vi "ConnectedStatusToSLServer.vi"() -> ()   [LabVIEW 2020]
doc: "This VI connects to the SystemLink server and writes two tag values: \nTrue to \"SERVER_NAME.System.Connected\"\nTimestamp of Start Time to \"SERVER_NAME.System.StartTime\""
uses:
  <vilib>/Skyline/Tag/Shared/typedefs/DataType.ctl
  StateStartTimeUpdate.ctl
  <vilib>/Skyline/Configuration/Configuration HTTP_class/NI Skyline Configuration HTTP.lvclass/NI Skyline Configuration HTTP.ctl
  <vilib>/Skyline/Configuration/Configuration HTTP_class/Open Configuration HTTP.vi
  <vilib>/Skyline/Configuration/HTTP/Open Configuration (Desktop).vi
  <vilib>/Skyline/Tag/Wrapper/Wrapper HTTP_class/Open Tag HTTP.vi
  <vilib>/Skyline/Tag/Wrapper/Wrapper_class/Write Tag (Boolean).vi
  <vilib>/Skyline/Tag/Wrapper/Wrapper_class/Delete Tag (Single).vi
  <vilib>/Skyline/Tag/Wrapper/Wrapper_class/Write Tag (Timestamp).vi
  <vilib>/nisyscfg/Close (System).vi
  <vilib>/Skyline/Configuration/Configuration HTTP_class/NI Skyline Configuration HTTP.lvclass
  <vilib>/Skyline/Configuration/Configuration_class/NI Skyline Configuration.lvclass
  <vilib>/Skyline/Tag/Wrapper/Wrapper_class/NI Skyline Tag.lvclass
  <vilib>/Skyline/Tag/Wrapper/Wrapper HTTP_class/NI Skyline Tag HTTP.lvclass
  <vilib>/Skyline/Tag/Shared/NI Skyline Tag.lvlib
  <vilib>/Skyline/Utilities/NI Skyline Utilities.lvlib
  <vilib>/nisyscfg/nisyscfg.lvlib
  <resource>/objmgr/nisysapi.rc
panel:
  in  "stop":bool
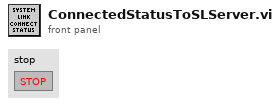
[diagram p1: front panel]
types:
  T1 = typedef "StateStartTimeUpdate.ctl" = enum16{"Init", "UpdateStartTime", "CleanUp"}
  T2 = typedef "NI Skyline Tag.lvlib/DataType.ctl" = enum32{"Double", "I32", "String", "Boolean", "U64", "Timestamp"}
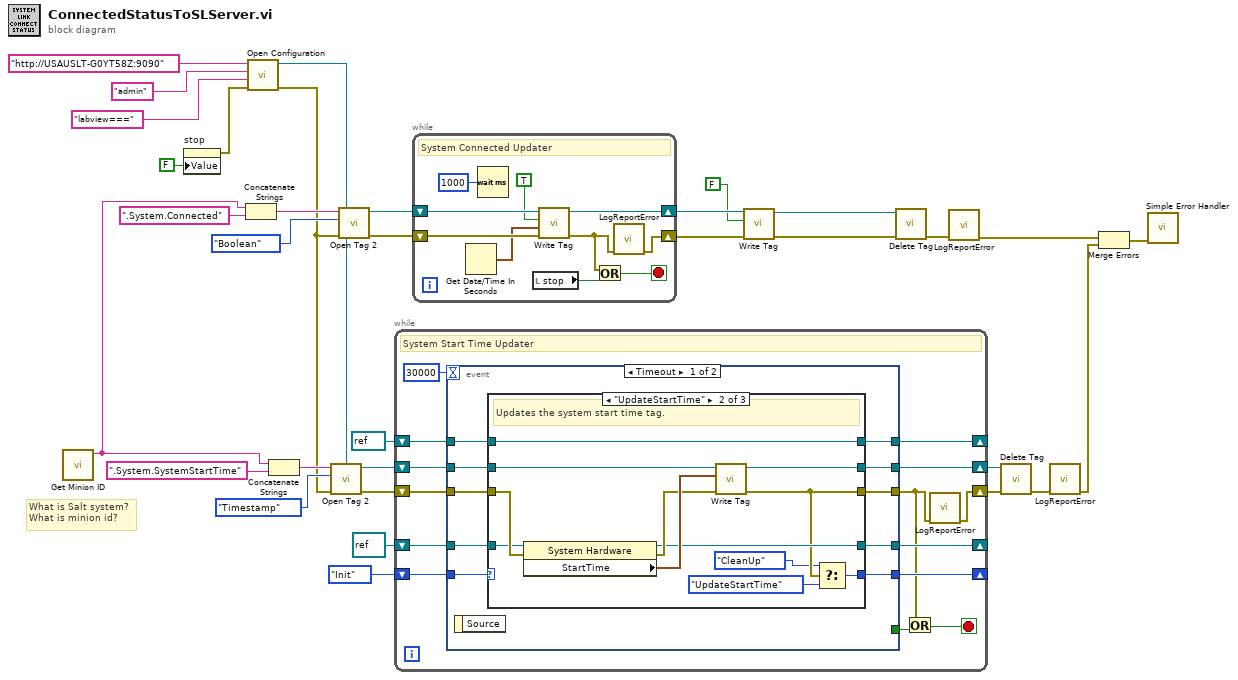
[diagram p0: block diagram]
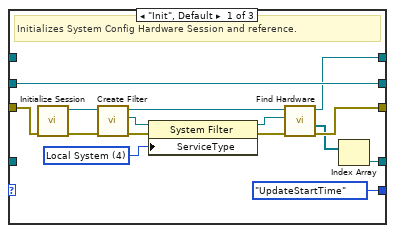
[diagram p2: hidden frame]
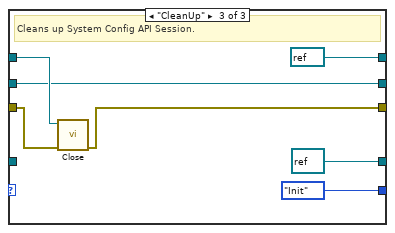
[diagram p3: hidden frame]
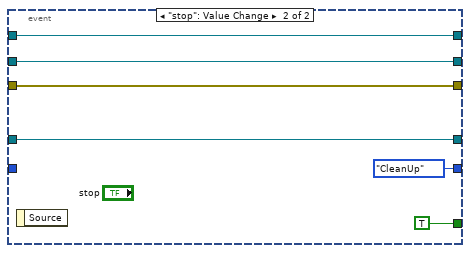
[diagram p4: hidden frame]
diagram:
  # "What is Salt system?\nWhat is minion id?"
  n1 = call <vilib>:"Get Minion ID.vi"() -> ("minion id"=w7:string)  [unwired: 11 in]
  n2 = property on="stop" class="Bool (strict)"("Value"=FALSE ("stop")) -> (error out=w8:errorcluster)  [unwired: 2 in, 1 out]
  n3 = Concatenate Strings(w7, ".System.Connected" ("path")) -> (w10:string)
  n4 = call-poly <vilib>:"Open Configuration.vi"("error in (no error)"=w8, "password"="labview===", "username"="admin", "server url"="http://USAUSLT-G0YT58Z:9090") -> ("error out"=w6:errorcluster, "configuration"=w9:refnum<class "NI Skyline Configuration HTTP.lvclass">)  [unwired: 6 in]
  n5 = Concatenate Strings(w7, ".System.SystemStartTime" ("path")) -> (w11:string)
  n6 = call-poly <vilib>:"Open Tag 2.vi"("configuration"=w9, "error in (no error)"=w6, "Data Type"=DataType."Timestamp", "path"=w11) -> ("error out"=w20:errorcluster, "tag"=w21:refnum<class "NI Skyline Tag.lvclass">)  [unwired: 6 in]
  n7 = call-poly <vilib>:"Open Tag 2.vi"("configuration"=w9, "error in (no error)"=w6, "Data Type"=DataType."Boolean", "path"=w10) -> ("error out"=w28:errorcluster, "tag"=w14:refnum<class "NI Skyline Tag.lvclass">)  [unwired: 6 in]
  n8 = while {
    shift-right: [w46] -> w19
    shift-left: w21 -> [w47]
    shift-right: [w35] -> w18
    shift-left: w20 -> [w45]
    shift-right: [w43] -> _
    shift-left: refnum<k20> refnum ("resource out") -> [w41]
    shift-right: [w42] -> _
    shift-left: StateStartTimeUpdate."Init" -> [w44]
    shift-right: [w40] -> _
    shift-left: refnum<k21> refnum ("Session out") -> [w39]
    stop <- w38 stop-if-true
    # "System Start Time Updater"
    n9 = event shown="[0] Timeout" {
      selector: _ -> [_ _]
      dyn-events: _ -> [_ _]
      timeout: u32 30000 ("milliseconds to wait") -> [_ _]
      tunnel: w47 -> [w57 w93]
      tunnel: [w56 w93] -> w46
      tunnel: [w55 w92] -> w34
      tunnel: w45 -> [w54 w92]
      tunnel: w44 -> [w53 _]
      tunnel: [w52 w96] -> w43
      tunnel: [w51 StateStartTimeUpdate."CleanUp"] -> w42
      tunnel: w41 -> [w50 w96]
      tunnel: [w49 w94] -> w40
      tunnel: w39 -> [w48 w94]
      tunnel: [_ TRUE ("stop")] -> w36
      event Timeout {
        n10 = event-data() -> ()  [unwired: 1 in, 1 out]
        n11 = case shown="\"UpdateStartTime\"" w53 {
          tunnel: w57 -> [w72 w84 w88]
          tunnel: [w72 w83 w88] -> w56
          tunnel: [w62 w76 w86] -> w55
          tunnel: w54 -> [w71 w81 w90]
          tunnel: [w60 w78 refnum<k20> refnum ("resource out")] -> w52
          tunnel: [StateStartTimeUpdate."UpdateStartTime" w74 StateStartTimeUpdate."Init"] -> w51
          tunnel: w50 -> [_ w79 _]
          tunnel: [w58 w77 refnum<k21> refnum ("Session out")] -> w49
          tunnel: w48 -> [_ w77 w91]
          frame "Init", Default {
            w66 = u32 4 items=["NI Network Resource", "NI Real-Time", "NI System Configuration", "NI Web Interface", "Local System", "Local Network Adapter", "Local Time Keeper", "Local Time Reference", "LXI Instrument", "Local FPGA"] ("Service Type")
            # "Initializes System Config Hardware Session and reference."
            n12 = call <vilib>:"Initialize Session.vi"("error in (no error)"=w71) -> ("error out"=w67:errorcluster, "Session out"=w68:refnum<k21>)  [unwired: 9 in]
            n13 = call <vilib>:"Create Filter.vi"("error in (no error)"=w67, "Session in"=w68) -> ("error out"=w69:errorcluster, "Filter out"=w70:refnum<k20>, "Session out"=w63:refnum<k21>)  [unwired: 7 in]
            n14 = property class="System Filter"(reference=w70, error in=w69, "ServiceType"=w66) -> (reference out=w65:refnum<k20>, error out=w64:errorcluster)
            n15 = call <vilib>:"Find Hardware.vi"("error in (no error)"=w64, "Filter in"=w65, "Session in"=w63) -> ("error out"=w62:errorcluster, "Resources out"=w61:refnum<k20>[], "Session out"=w58:refnum<k21>)  [unwired: 5 in, 1 out]
            n16 = Index Array(array=w61) -> (element=w60:refnum<k20>)  [unwired: 1 in]
          }
          frame "UpdateStartTime" {
            # "Updates the system start time tag."
            n17 = property class="System Hardware"(reference=w79, error in=w81) -> (reference out=w78:refnum<k20>, error out=w80:errorcluster, "StartTime"=w82:timestamp)
            n18 = call-poly <vilib>:"Write Tag.vi"("error in (no error)"=w80, "value"=w82, "tag in"=w84) -> ("error out"=w76:errorcluster, "tag out"=w83:refnum<class "NI Skyline Tag.lvclass">)  [unwired: 7 in]
            n19 = Select(t=StateStartTimeUpdate."CleanUp", s=w76, f=StateStartTimeUpdate."UpdateStartTime") -> (s? t:f=w74:T1)
          }
          frame "CleanUp" {
            # "Cleans up System Config API Session."
            n20 = call-poly <vilib>:"Close.vi"("error in (no error)"=w90, "Session in"=w91) -> ("error out"=w86:errorcluster)  [unwired: 9 in]
          }
        }
      }
      event "stop": Value Change {
        n21 = event-data() -> ()  [unwired: 1 in, 1 out]
      }
    }
    n22 = Or(x=w34, y=w36) -> (x .or. y?=w38:bool)
    n23 = call "LogReportError.vi"("error in (no error)"=w34) -> ("error out"=w35:errorcluster)  [unwired: 10 in]
  }
  n24 = while {
    shift-right: [w99] -> w26
    shift-left: w28 -> [w106]
    shift-right: [w105] -> w27
    shift-left: w14 -> [w107]
    stop <- w101 stop-if-true
    # "System Connected Updater"
    n25 = Get Date/Time In Seconds() -> (seconds since 1Jan1904=w103:timestamp)
    n26 = Wait (ms)(milliseconds to wait=u32 1000) -> ()  [unwired: 1 out]
    n27 = local read "stop"() -> (w100:bool)
    n28 = call-poly <vilib>:"Write Tag.vi"("error in (no error)"=w106, "time stamp"=w103, "value"=TRUE, "tag in"=w107) -> ("error out"=w98:errorcluster, "tag out"=w105:refnum<class "NI Skyline Tag.lvclass">)  [unwired: 6 in]
    n29 = Or(x=w98, y=w100) -> (x .or. y?=w101:bool)
    n30 = call "LogReportError.vi"("error in (no error)"=w98) -> ("error out"=w99:errorcluster)  [unwired: 10 in]
  }
  n31 = call-poly <vilib>:"Write Tag.vi"("error in (no error)"=w26, "value"=FALSE, "tag in"=w27) -> ("error out"=w23:errorcluster, "tag out"=w24:refnum<class "NI Skyline Tag.lvclass">)  [unwired: 7 in]
  n32 = call-poly <vilib>:"Delete Tag.vi"("error in (no error)"=w23, "tag"=w24) -> ("error out"=w4:errorcluster)  [unwired: 9 in]
  n33 = call "LogReportError.vi"("error in (no error)"=w4) -> ("error out"=w3:errorcluster)  [unwired: 10 in]
  n34 = call-poly <vilib>:"Delete Tag.vi"("error in (no error)"=w18, "tag"=w19) -> ("error out"=w2:errorcluster)  [unwired: 9 in]
  n35 = call "LogReportError.vi"("error in (no error)"=w2) -> ("error out"=w1:errorcluster)  [unwired: 10 in]
  n36 = Merge Errors(w3, w1) -> (w5:errorcluster)
  n37 = call <vilib>:"Simple Error Handler.vi"("error in (no error)"=w5) -> ()  [unwired: 4 in, 5 out]
